vi "Servo Control.vi"(10 "Position":dbl, 11 "Enum":T1) -> ()   [LabVIEW 2014]
uses:
  SRE Enum.ctl
  Text Variable VIs/Read Number Variable.vi
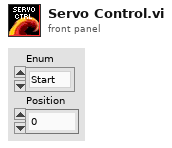
[diagram p1: front panel]
types:
  T1 = typedef "SRE Enum.ctl" = enum16{"Start", "Run", "End"}
  T2 = typedef "WPI_ServoDeviceRef.ctl" = cluster{"DeviceStatus":errorcluster, "Controller":T3, "PWM Channel":T4, "DeadBand":T5}
  T3 = typedef "FPGA_TypedefDigitalModule.ctl" = enum16{"Controller 1"}
  T4 = typedef "FPGA_DIOPWMChannel.ctl" = enum8{"PWM 0", "PWM 1", "PWM 2", "PWM 3", "PWM 4", "PWM 5", "PWM 6", "PWM 7", "PWM 8", "PWM 9", "PWM MXP 0", "PWM MXP 1", "PWM MXP 2", "PWM MXP 3", "PWM MXP 4", "PWM MXP 5", "PWM MXP 6", "PWM MXP 7", "PWM MXP 8", "PWM MXP 9", "Invalid"}
  T5 = typedef "WPI_PWMDeadband.ctl" = cluster{"Name":string, "maxPositivePwm":i32, "minPositivePwm":i32, "centerPwm":i32, "maxNegativePwm":i32, "minNegativePwm":i32, "angularRange":u16}
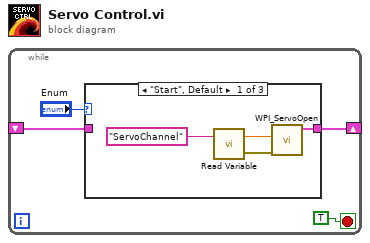
[diagram p0: block diagram]
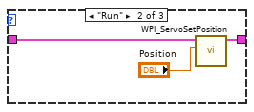
[diagram p2: hidden frame]
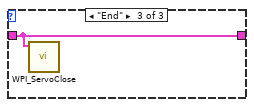
[diagram p3: hidden frame]
diagram:
  n1 = while {
    shift-right: [w2] -> _
    shift-left: _ -> [w1]
    stop <- TRUE stop-if-true
    n2 = case shown="\"Start\", Default" "Enum" {
      tunnel: [w5 w10 w12] -> w2
      tunnel: w1 -> [_ w11 w12]
      frame "Start", Default {
        n3 = call-poly "Read Variable.vi"("Name"="ServoChannel") -> ("error out"=w6:errorcluster, "number"=w8:dbl)  [unwired: 1 in]
        n4 = call <vilib>:"WPI_ServoOpen.vi"("error in (no error)"=w6, "PWM Channel"=w8) -> ("ServoDeviceRef"=w5:T2)  [unwired: 8 in, 1 out]
      }
      frame "Run" {
        n5 = call <vilib>:"WPI_ServoSetPosition.vi"("Position"="Position", "ServoDeviceRef"=w11) -> ("ServoDeviceRef"=w10:T2)  [unwired: 8 in, 1 out]
      }
      frame "End" {
        n6 = call <vilib>:"WPI_ServoClose.vi"("MotorControlDevRef"=w12) -> ()  [unwired: 10 in, 1 out]
      }
    }
  }
